vi "DW Test Copy.vi"(0 "inputEnum1":u32(ring)=1 items=["kType"=1, "uType"=2], 1 "outputEnum1":u32(ring)=1 items=["kType"=1, "uType"=2], 2 "inputEnum2":u32(ring)=3 items=["iType"=3, "jType"=4], 3 "outputEnum2":u32(ring)=3 items=["iType"=3, "jType"=4], 4 "runtimeSize":u32, 5 "inputRunTimeSizeArray":i32[](array[numeric])=array[4097 elements], 6 "outputRunTimeSizeArray":i32[](array[numeric])=array[4097 elements], 8 "inputBool":bool, 9 "outputBool":bool, 10 "inputString":string, 11 "outputString":string, 12 "left":i32, 13 "top":i32, 14 "outputStruct":cluster{"left":i32, "top":i32}) -> (17 "outputString out":string, 19 "outputBool out":bool, 20 "outputStruct out":cluster{"left":i32, "top":i32}, 21 "outputEnum1 out":u32(ring)=1 items=["kType"=1, "uType"=2], 23 "outputEnum2 out":u32(ring)=3 items=["iType"=3, "jType"=4], 25 "inputRunTimeSizeArray out":i32[](array[numeric]), 26 "outputRunTimeSizeArray out":i32[](array[numeric]))   [LabVIEW 2020, in "ImportSharedLibraryExample.lvlib"]
doc: "void DWTest_Copy(MyEnum inputEnum1, \n MyEnum* outputEnum1, \n enum YourEnum inputEnum2, \n enum YourEnum* outputEnum2,\n unsigned int runtimeSize, \n int inputRunTimeSizeArray[], \n int outputRunTimeSizeArray[],\n bool inputBool, \n bool* outputBool,\n const char inputString[], \n char outputString[],\n StructWithOnlyIntElement inputStruct, \n StructWithOnlyIntElement* outputStruct);"
uses:
  ImportSharedLibraryExample.lvlib
  ImportSharedLibraryExample.dll
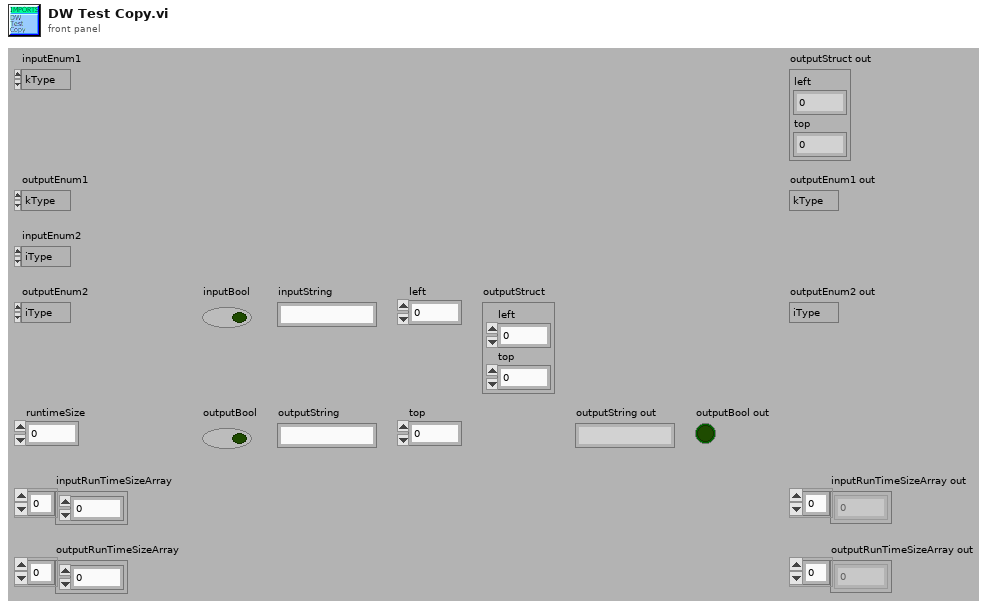
[diagram p1: front panel]
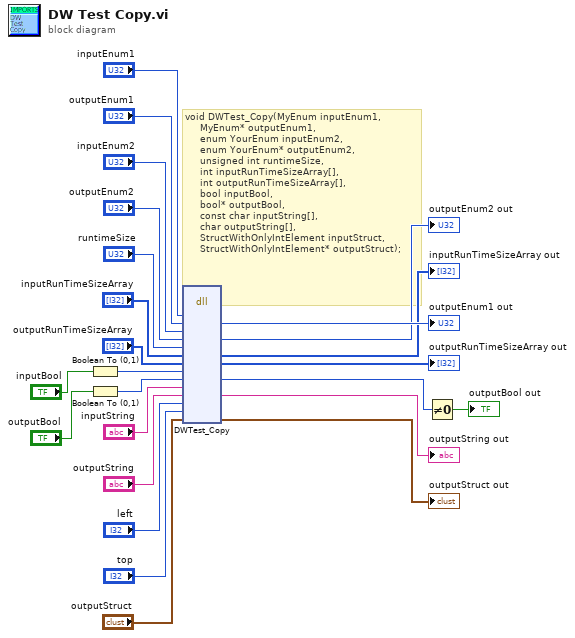
[diagram p0: block diagram]
diagram:
  # "void DWTest_Copy(MyEnum inputEnum1, \n     MyEnum* outputEnum1, \n     enum YourEnum inputEnum2, \n     enum YourEnum* outputEnum2,\n     unsigned int runtimeSize, \n     int inputRunTimeSizeArray[], \n     int outputRunTimeSizeArray[],\n     bool inputBool, \n     bool* outputBool,\n     const char inputString[], \n     char outputString[],\n     StructWithOnlyIntElement inputStruct, \n     StructWithOnlyIntElement* outputStruct);"
  n1 = Boolean To (0,1)(Boolean="inputBool") -> (0, 1=w12:i16)
  n2 = Boolean To (0,1)(Boolean="outputBool") -> (0, 1=w10:i16)
  n3 = dll-call lib="e:/builds/penguin/labview/branches/2020/dev/dist/examples/dll/ImportSharedLibraryExample/ImportSharedLibraryExample.*" fn="DWTest_Copy"("inputEnum1"="inputEnum1", "outputEnum1"="outputEnum1", "inputEnum2"="inputEnum2", "outputEnum2"="outputEnum2", "runtimeSize"="runtimeSize", "inputRunTimeSizeArray"="inputRunTimeSizeArray", "outputRunTimeSizeArray"="outputRunTimeSizeArray", "inputBool"=w12, "outputBool"=w10, "inputString"="inputString", "outputString"="outputString", "left"="left", "top"="top", "outputStruct"="outputStruct") -> ("outputEnum1"=→"outputEnum1 out":u32, "outputEnum2"=→"outputEnum2 out":u32, "inputRunTimeSizeArray"=→"inputRunTimeSizeArray out":i32[], "outputRunTimeSizeArray"=→"outputRunTimeSizeArray out":i32[], "outputBool"=w8:u8, "outputString"=→"outputString out":string, "outputStruct"=→"outputStruct out":cluster{"left":i32, "top":i32})  [unwired: 9 in, 4 out]
  n4 = Not Equal To 0?(x=w8) -> (x != 0?=→"outputBool out":bool)
